vi "Clamp.vi"(7 "Model Name":T1, 8 "Error In":errorcluster, 9 "Intialize?":bool=TRUE, 10 "Inputs":T2) -> (0 "error out":errorcluster, 1 "Completed":bool, 4 "Status":cluster{"Status":string, "Elapsed Time":dbl})   [LabVIEW 2017]
uses:
  controls/All Inputs.ctl
  controls/SACB DI.ctl
  controls/Model Name.ctl
  controls/Clamp.ctl
  controls/FGV DO.ctl
panel:
  in  "Delay (for Clamp)":u32
  in  "Timeout (ms)":u32=15000
  # "Inputs"
  # "Variables"
  # "Outputs"
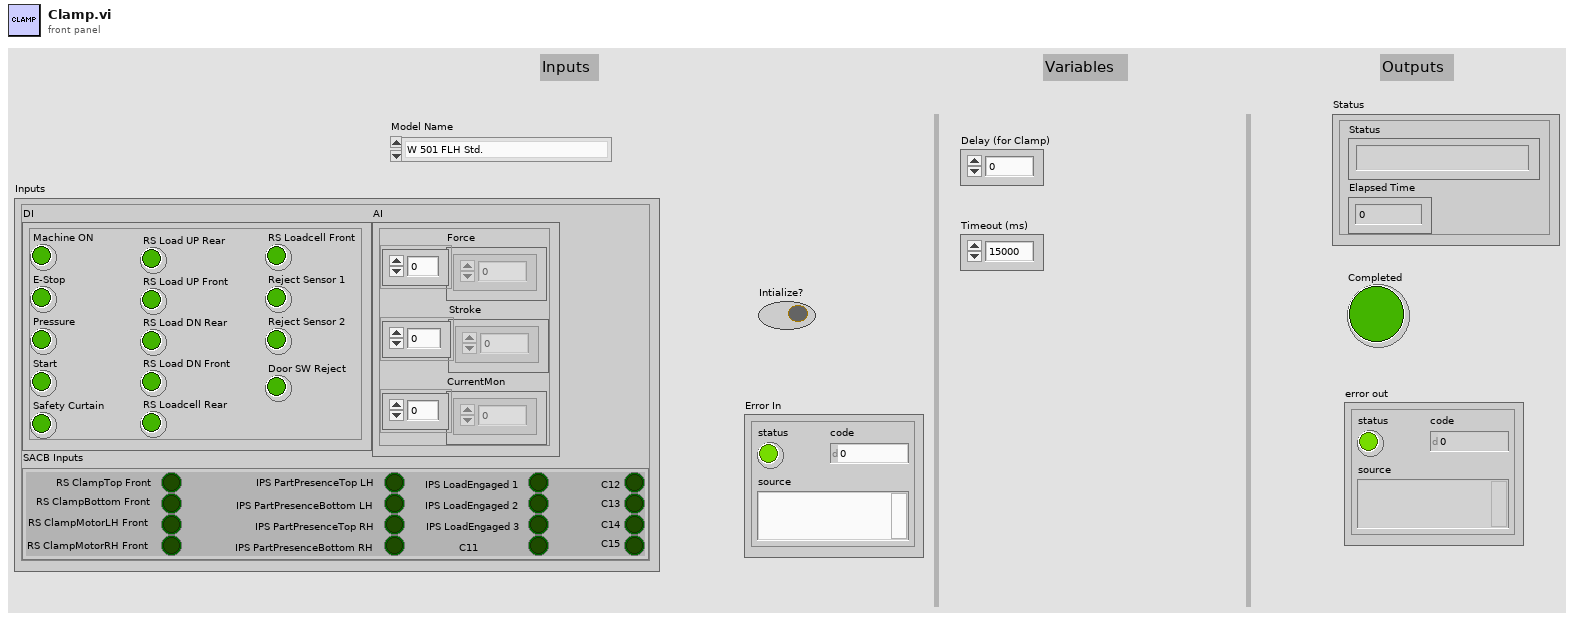
[diagram p1: front panel]
types:
  T1 = typedef "Model Name.ctl" = enum16{"W 501 FLH Std.", "W 501 FRH Std.", "W 601 FR RH Std", "W 601 FR LH Std", "W 601 RR RH Std", "W 601 RR LH Std", "W 601 FR RH AP", "W 601 FR LH AP", "W 601 RR RH AP", "W 601 RR LH AP"}
  T2 = typedef "All Inputs.ctl" = cluster{"DI":cluster{"Machine ON":bool, "E-Stop":bool, "Pressure":bool, "Start":bool, "Safety Curtain":bool, "RS Load UP Rear":bool, "RS Load UP Front":bool, "RS Load DN Rear":bool, "RS Load DN Front":bool, "RS Loadcell Rear":bool, "RS Loadcell Front":bool, "Reject Sensor 1":bool, "Reject Sensor 2":bool, "Door SW Reject":bool}, "AI":cluster{"Force":dbl[], "Stroke":dbl[], "CurrentMon":dbl[]}, "SACB Inputs":T3}
  T3 = typedef "SACB DI.ctl" = cluster{"RS ClampTop Front":bool, "RS ClampBottom Front":bool, "RS ClampMotorLH Front":bool, "RS ClampMotorRH Front":bool, "IPS PartPresenceTop LH":bool, "IPS PartPresenceBottom LH":bool, "IPS PartPresenceTop RH":bool, "IPS PartPresenceBottom RH":bool, "IPS LoadEngaged 1":bool, "IPS LoadEngaged 2":bool, "IPS LoadEngaged 3":bool, "C11":bool, "C12":bool, "C13":bool, "C14":bool, "C15":bool}
  T4 = typedef "Clamp.ctl" = enum16{"Initialize", "Engage Clamping", "Delay (for Clamp)", "Done", "Error"}
  T5 = typedef "FGV DO.ctl" = enum16{"Initialize", "Start Task", "Clamping", "Load CYL", "Contactors", "Loadcell CYL", "BSL", "Read DO", "Clear Tasks", "Clear Task"}
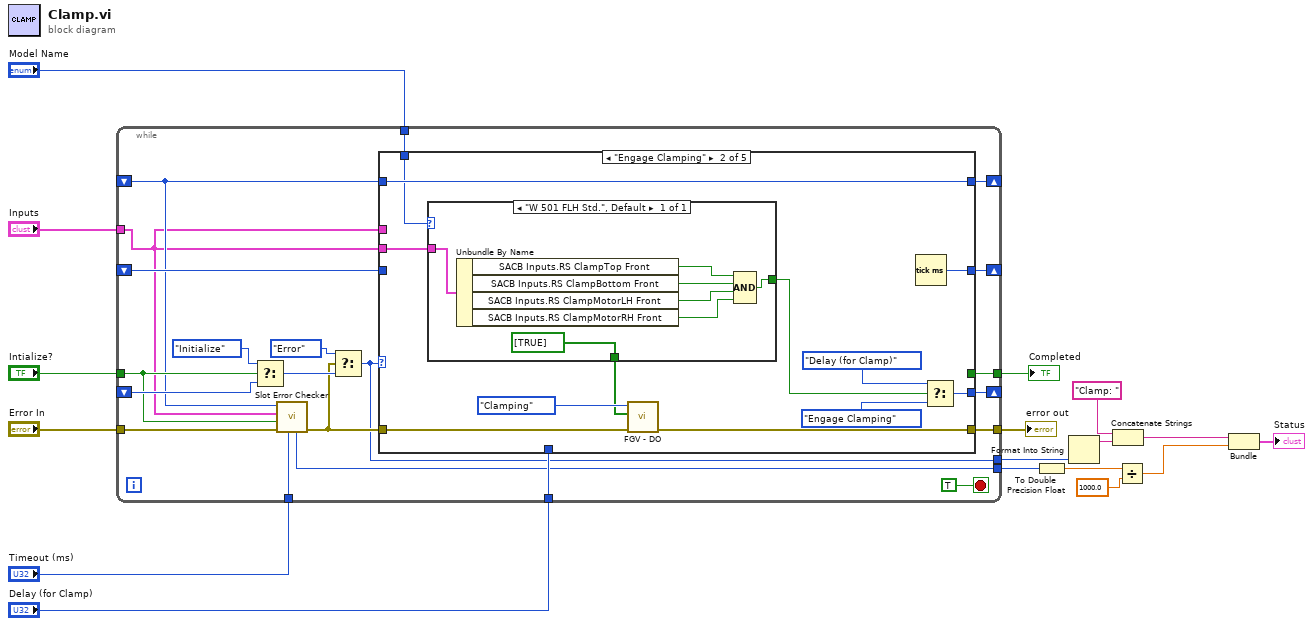
[diagram p0: block diagram]
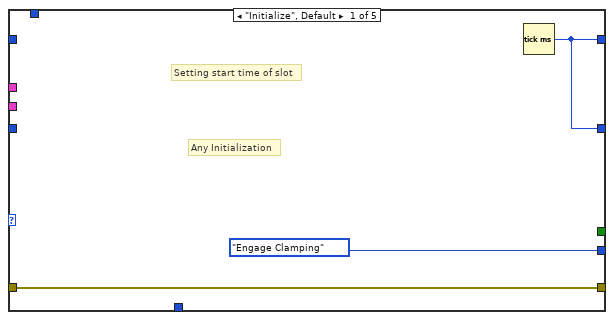
[diagram p2: hidden frame]
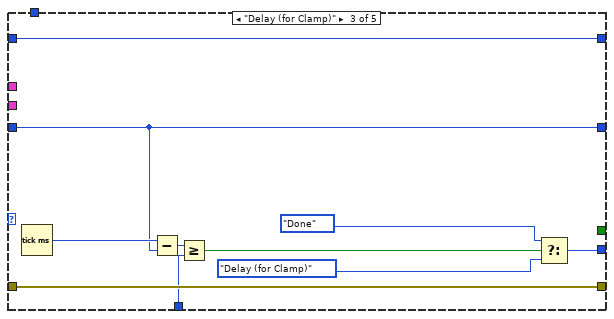
[diagram p3: hidden frame]
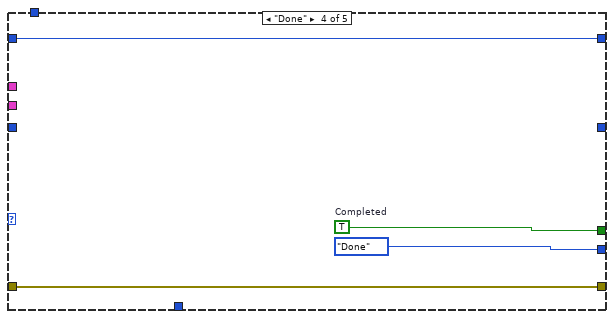
[diagram p4: hidden frame]
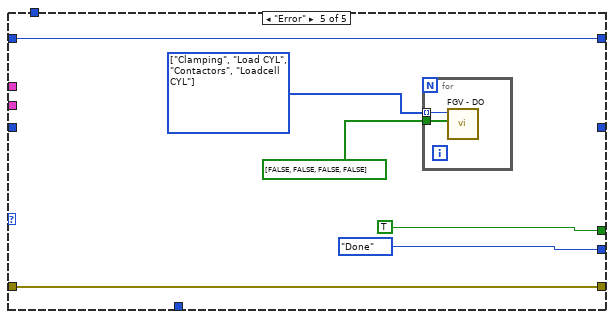
[diagram p5: hidden frame]
diagram:
  n1 = while {
    tunnel: "Intialize?" -> [w28]
    shift-right: [w35] -> _
    shift-left: _ -> [w37]
    shift-right: [w34] -> _
    shift-left: _ -> [w33]
    tunnel: "Error In" -> [w29]
    tunnel: [w32] -> w17
    tunnel: [w31] -> w16
    tunnel: "Inputs" -> [w18]
    shift-right: [w30] -> _
    shift-left: _ -> [w27]
    tunnel: "Delay (for Clamp)" -> [w23]
    tunnel: "Timeout (ms)" -> [w22]
    tunnel: [w21] -> w3
    tunnel: [w20] -> w2
    tunnel: "Model Name" -> [w19]
    stop <- TRUE stop-if-true
    n2 = Select(t=Clamp."Initialize", s=w28, f=w37) -> (s? t:f=w26:T4)
    n3 = call "Slot Error Checker.vi"("Timeout (ms)"=w22, "error in (no error)"=w29, "Intialize?"=w28, "Inputs"=w18, "start time"=w27) -> ("error out"=w25:errorcluster, "Slot Time"=w21:u32)  [unwired: 4 in, 1 out]
    n4 = Select(t=Clamp."Error", s=w25, f=w26) -> (s? t:f=w20:T4)
    n5 = case shown="\"Engage Clamping\"" w20 {
      tunnel: [Clamp."Engage Clamping" w45 w67 Clamp."Done" Clamp."Done"] -> w35
      tunnel: [w39 w50 w69 _ _] -> w34
      tunnel: w33 -> [_ _ w69 _ _]
      tunnel: w25 -> [w40 w53 w65 w73 w80]
      tunnel: [w40 w52 w65 w73 w80] -> w32
      tunnel: [_ _ _ w72 TRUE ("Completed")] -> w31
      tunnel: w18 -> [_ _ _ _ _]
      tunnel: [w39 w49 w62 w71 w77] -> w30
      tunnel: w27 -> [_ w49 w62 w71 w77]
      tunnel: w23 -> [_ _ w61 _ _]
      tunnel: w19 -> [_ w48 _ _ _]
      tunnel: w18 -> [_ w46 _ _ _]
      frame "Initialize", Default {
        # "Setting start time of slot"
        # "Any Initialization"
        n6 = Tick Count (ms)() -> (millisecond timer value=w39:u32)
      }
      frame "Engage Clamping" {
        n7 = case shown="\"W 501 FLH Std.\", Default" w48 {
          tunnel: [bool[] [TRUE] ("Digital Outs")] -> w47
          tunnel: w46 -> [w56]
          tunnel: [w57] -> w42
          frame "W 501 FLH Std.", Default {
            n8 = Unbundle By Name(w56) -> ("SACB Inputs.RS ClampTop Front"=w58:bool, "SACB Inputs.RS ClampBottom Front"=w59:bool, "SACB Inputs.RS ClampMotorLH Front"=w55:bool, "SACB Inputs.RS ClampMotorRH Front"=w54:bool)
            n9 = Compound Arithmetic op=AND(w58, w59, w55, w54) -> (w57:bool)
          }
        }
        n10 = call "FGV - DO.vi"("error in"=w53, "Digital Outs"=w47, "State"=FGV_DO."Clamping") -> ("error out"=w52:errorcluster)  [unwired: 7 in, 1 out]
        n11 = Tick Count (ms)() -> (millisecond timer value=w50:u32)
        n12 = Select(t=Clamp."Delay (for Clamp)", s=w42, f=Clamp."Engage Clamping") -> (s? t:f=w45:T4)
      }
      frame "Delay (for Clamp)" {
        n13 = Tick Count (ms)() -> (millisecond timer value=w70:u32)
        n14 = Subtract(x=w70, y=w69) -> (x-y=w68:u32)
        n15 = Greater Or Equal?(x=w68, y=w61) -> (x >= y?=w66:bool)
        n16 = Select(t=Clamp."Done", s=w66, f=Clamp."Delay (for Clamp)") -> (s? t:f=w67:T4)
      }
      frame "Done" {
        w72 = TRUE  # Completed
      }
      frame "Error" {
        w75 = T5[] [enum."Clamping", enum."Load CYL", enum."Contactors", enum."Loadcell CYL"] items=["Initialize", "Start Task", "Clamping", "Load CYL", "Contactors", "Loadcell CYL", "BSL", "Read DO", "Clear Tasks", "Clear Task"]
        n17 = for {
          tunnel: w75 -> [w82] mode=indexing
          tunnel: bool[] [FALSE, FALSE, FALSE, FALSE] ("Digital Outs") -> [w81]
          n18 = call "FGV - DO.vi"("Digital Outs"=w81, "State"=w82) -> ()  [unwired: 8 in, 2 out]
        }
      }
    }
  }
  "error out" <- w17
  "Completed" <- w16
  n19 = To Double Precision Float(number=w3) -> (double precision float=w8:dbl)
  n20 = Format Into String(w2) -> (resulting string=w10:string)  [unwired: 3 in, 1 out]
  n21 = Concatenate Strings("Clamp: ", w10) -> (w6:string)
  n22 = Divide(x=w8, y=1000.0) -> (x/y=w5:dbl)
  n23 = Bundle(w6, w5) -> (→"Status":cluster{string, dbl})  [unwired: 1 in]
